vi "Data Parsing2.vi"(5 "read buffer":string, 7 "All Data Elements (False)":bool, 11 "error in":errorcluster) -> (6 "Measurement Data":dbl[](array[numeric]), 8 "Time Stamp":string[](array[string]), 10 "Channel":string[](array[string]), 15 "Reading Number":string[](array[string]))   [LabVIEW 2015]
doc: "This subVI parses data read in from buffer."
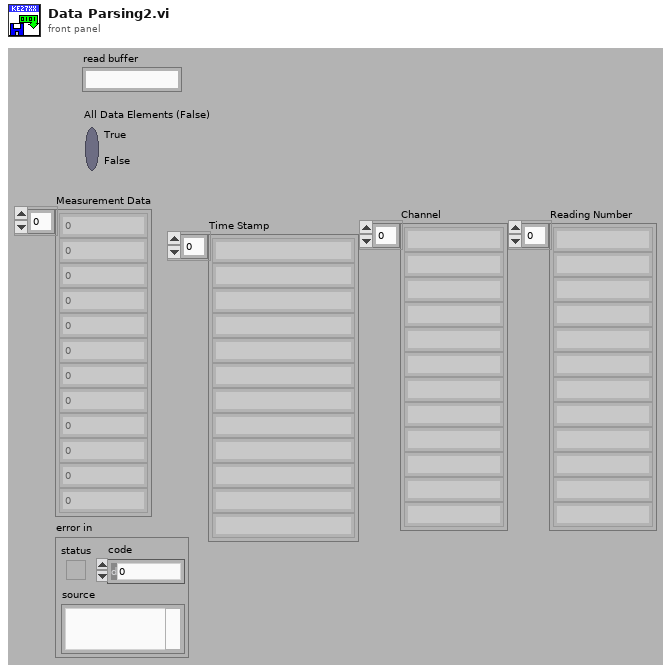
[diagram p1: front panel]
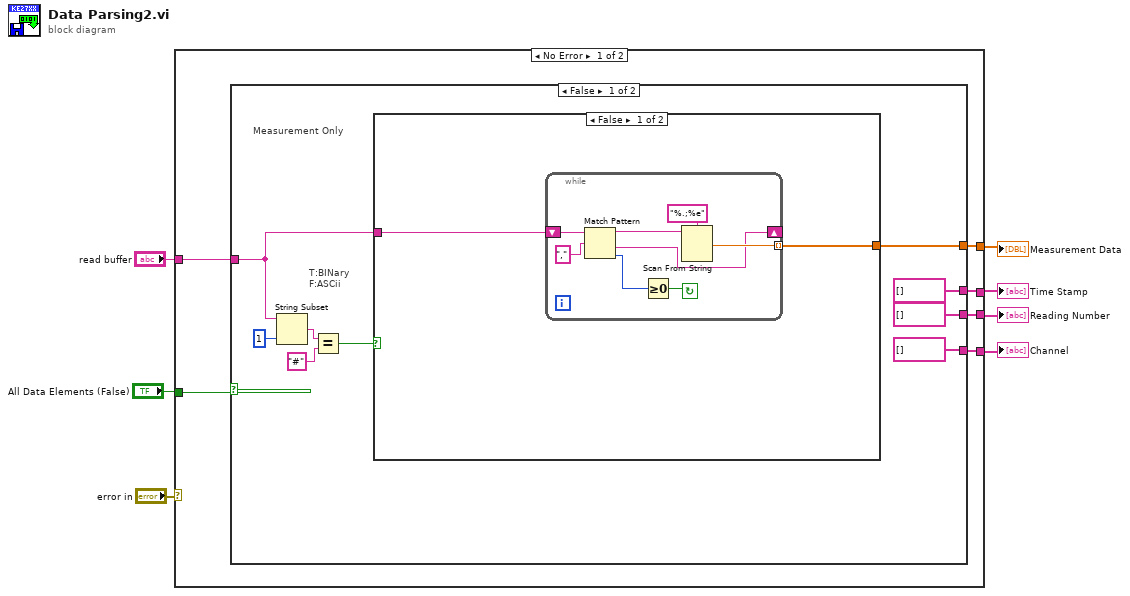
[diagram p0: block diagram]
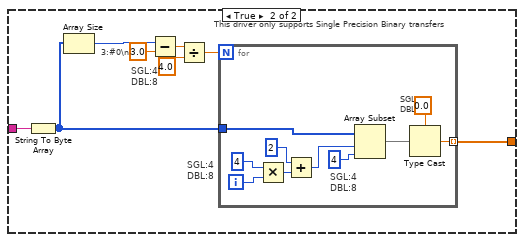
[diagram p2: hidden frame]
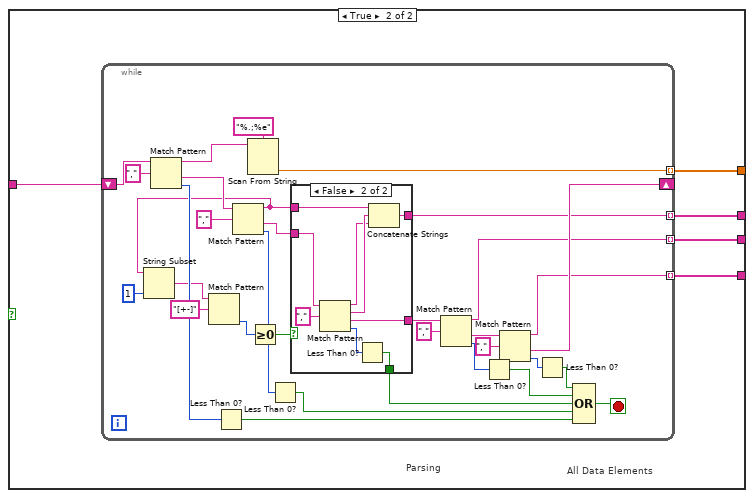
[diagram p3: hidden frame]
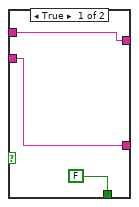
[diagram p4: hidden frame]
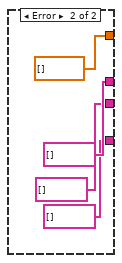
[diagram p5: hidden frame]
diagram:
  n1 = case shown="No Error" "error in" {
    tunnel: "All Data Elements (False)" -> [w13 _]
    tunnel: [w9 dbl[] []] -> w5
    tunnel: [w12 string[] []] -> w4
    tunnel: [w11 string[] []] -> w3
    tunnel: [w10 string[] []] -> w2
    tunnel: "read buffer" -> [w8 _]
    frame No Error {
      n2 = case shown="False" w13 {
        tunnel: [string[] [] w54] -> w12
        tunnel: [string[] [] w53] -> w11
        tunnel: [string[] [] w52] -> w10
        tunnel: [w15 w55] -> w9
        tunnel: w8 -> [w14 w51]
        frame False {
          # "T:BINary\nF:ASCii"
          # "Measurement Only"
          n3 = String Subset(string=w14, length (rest)=1 ("length (rest)")) -> (substring=w22:string)  [unwired: 1 in]
          n4 = Equal?(x=w22, y="#") -> (x = y?=w19:bool)
          n5 = case shown="False" w19 {
            tunnel: [w24 w34] -> w15
            tunnel: w14 -> [w23 w33]
            frame False {
              n6 = while {
                shift-right: [w25] -> _
                shift-left: w23 -> [w26]
                tunnel: [w28] -> w24 mode=indexing
                stop <- w31 continue-if-true
                n7 = Match Pattern(string=w26, regular expression="," ("search string/char (-)")) -> (before substring=w30:string, after substring=w25:string, offset past match=w27:i32)  [unwired: 1 in, 1 out]
                n8 = Greater Or Equal To 0?(x=w27) -> (x >= 0?=w31:bool)
                n9 = Scan From String(format string="%.;%e", input string=w30) -> (output 1=w28:dbl)  [unwired: 3 in, 3 out]
              }
            }
            frame True {
              # "This driver only supports Single Precision Binary transfers"
              # "3:#0\\n"
              # "SGL:4\nDBL:8"
              # "SGL:4\nDBL:8"
              n10 = String To Byte Array(string=w33) -> (unsigned byte array=w36:u8[])
              n11 = Array Size(array=w36) -> (size(s)=w40:i32)
              n12 = Subtract(x=w40, y=3.0) -> (x-y=w37:dbl)
              n13 = Divide(x=w37, y=4.0) -> (x/y=w35:dbl)
              n14 = for {
                N: w35 -> [_]
                tunnel: w36 -> [w42]
                tunnel: [w41] -> w34 mode=indexing
                i -> [w47]
                # "SGL\nDBL"
                # "SGL:4\nDBL:8"
                n15 = Multiply(x=4, y=w47) -> (x*y=w46:i32)
                n16 = Add(x=2, y=w46) -> (x+y=w43:i32)
                n17 = Array Subset(array=w42, index=w43, length=4) -> (w49:u8[])
                n18 = Type Cast(type=sgl 0.0, x=w49) -> (*(type *) &x=w41:sgl)
              }
            }
          }
        }
        frame True {
          # "All Data Elements"
          # "Parsing"
          n19 = while {
            shift-right: [w72] -> _
            shift-left: w51 -> [w83]
            tunnel: [w84] -> w55 mode=indexing
            tunnel: [w64] -> w54 mode=indexing
            tunnel: [w57] -> w52 mode=indexing
            tunnel: [w56] -> w53 mode=indexing
            stop <- w76 stop-if-true
            n20 = Match Pattern(string=w83, regular expression="," ("search string/char (-)")) -> (before substring=w86:string, after substring=w82:string, offset past match=w79:i32)  [unwired: 1 in, 1 out]
            n21 = Less Than 0?(x=w79) -> (x < 0?=w78:bool)
            n22 = Match Pattern(string=w82, regular expression="," ("search string/char (-)")) -> (before substring=w59:string, after substring=w70:string, offset past match=w80:i32)  [unwired: 1 in, 1 out]
            n23 = String Subset(string=w59, length (rest)=1 ("length (rest)")) -> (substring=w60:string)  [unwired: 1 in]
            n24 = Match Pattern(string=w60, regular expression="[+-]") -> (offset past match=w61:i32)  [unwired: 1 in, 3 out]
            n25 = Scan From String(format string="%.;%e", input string=w86) -> (output 1=w84:dbl)  [unwired: 3 in, 3 out]
            n26 = Greater Or Equal To 0?(x=w61) -> (x >= 0?=w62:bool)
            n27 = Less Than 0?(x=w80) -> (x < 0?=w77:bool)
            n28 = case shown="False" w62 {
              tunnel: [w89 w98] -> w69
              tunnel: [FALSE w96] -> w65
              tunnel: w70 -> [w89 w95]
              tunnel: w59 -> [w88 w94]
              tunnel: [w88 w91] -> w64
              frame True {
              }
              frame False {
                n29 = Match Pattern(string=w95, regular expression="," ("search string/char (-)")) -> (before substring=w92:string, match substring=w93:string, after substring=w98:string, offset past match=w97:i32)  [unwired: 1 in]
                n30 = Less Than 0?(x=w97) -> (x < 0?=w96:bool)
                n31 = Concatenate Strings(w94, w93, w92) -> (w91:string)
              }
            }
            n32 = Match Pattern(string=w69, regular expression="," ("search string/char (-)")) -> (before substring=w57:string, after substring=w68:string, offset past match=w67:i32)  [unwired: 1 in, 1 out]
            n33 = Less Than 0?(x=w67) -> (x < 0?=w66:bool)
            n34 = Match Pattern(string=w68, regular expression="," ("search string/char (-)")) -> (before substring=w56:string, after substring=w72:string, offset past match=w75:i32)  [unwired: 1 in, 1 out]
            n35 = Less Than 0?(x=w75) -> (x < 0?=w73:bool)
            n36 = Compound Arithmetic op=OR(w73, w66, w65, w77, w78) -> (w76:bool)
          }
        }
      }
    }
    frame Error {
    }
  }
  "Measurement Data" <- w5
  "Time Stamp" <- w4
  "Channel" <- w3
  "Reading Number" <- w2
